vi "Parameter Files Error Dialog.vi"(8 "error in (no error)":errorcluster, 10 "File Parameters":string[](array[string]), 11 "SDF Parameters":string[](array[string])) -> (0 "error out":errorcluster)   [LabVIEW 2016, in "System Mapping Tool.lvlib"]
uses:
  System Mapping Tool.lvlib
panel:
  in  "OK":bool
  in  "Table Control":string[][](table)
  # "The following parameters referenced in the selected file were not found in the loaded system definition:"
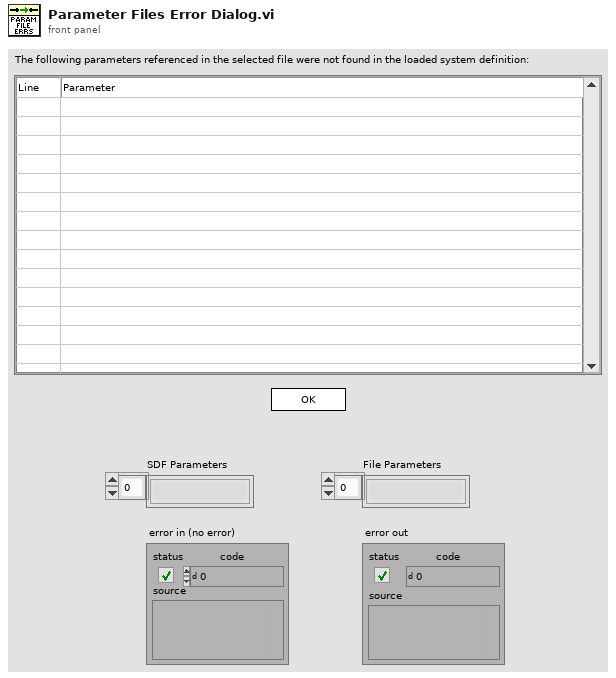
[diagram p1: front panel]
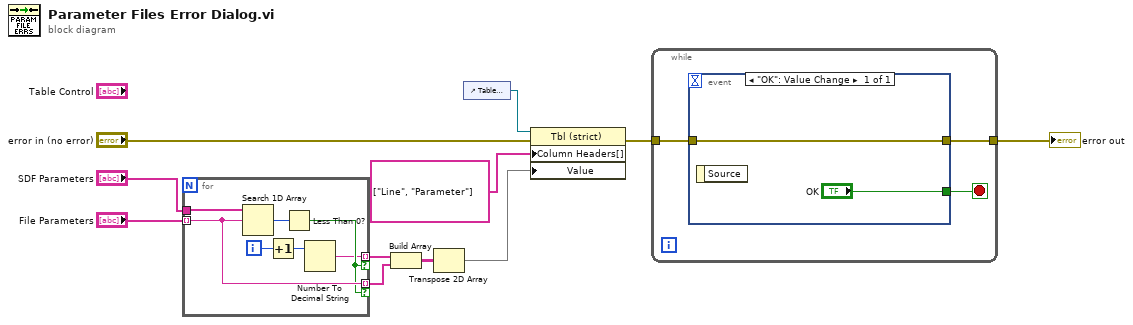
[diagram p0: block diagram]
diagram:
  n1 = for {
    tunnel: "File Parameters" -> [w16] mode=indexing
    tunnel: "SDF Parameters" -> [w18]
    tunnel: [w16] -> w1 mode=indexing if=w15
    tunnel: [w12] -> w2 mode=indexing if=w15
    i -> [w14]
    n2 = Search 1D Array(1D array=w18, element=w16) -> (index of element=w17:i32)  [unwired: 1 in]
    n3 = Increment(x=w14) -> (x+1=w13:i32)
    n4 = Less Than 0?(x=w17) -> (x < 0?=w15:bool)
    n5 = Number To Decimal String(number=w13) -> (decimal integer string=w12:string)  [unwired: 1 in]
  }
  n6 = Build Array(w2, w1) -> (w3:string[][])
  n7 = Transpose 2D Array(2D array=w3) -> (transposed array=w5:string[][])
  n8 = control-ref of="Table Control"() -> (w11:refnum<vi>)
  n9 = property class="Tbl (strict)"(reference=w11, error in="error in (no error)", "Column Headers[]"=string[] ["Line", "Parameter"], "Value"=w5) -> (error out=w8:errorcluster)  [unwired: 1 out]
  n10 = while {
    tunnel: [w20] -> w9
    tunnel: w8 -> [w19]
    stop <- w21 stop-if-true
    n11 = event shown="[0] \"OK\": Value Change" {
      selector: _ -> [_]
      dyn-events: _ -> [_]
      timeout: _ -> [_]
      tunnel: ["OK"] -> w21
      tunnel: [w22] -> w20
      tunnel: w19 -> [w22]
      event "OK": Value Change {
        n12 = event-data() -> ()  [unwired: 1 in, 1 out]
      }
    }
  }
  "error out" <- w9
